vi "Main.vi"(11 "Module Admin":refnum<class "Delacor_lib_QMH_Module Admin.lvclass">) -> ()   [LabVIEW 2020, in "FileIO.lvlib"]
doc: "This template is based off of the Queued Message Handler design pattern and the Queued Message Handler project template that ships with LabVIEW.\n\nThe main difference is that the queue is private to this module and communication between modules is performed via Broadcast and Request events.\n\nRequest events are wrapped in public API methods and are handled in the Event Handling Loop (EHL) of this VI. Any module can register for Broadcast events sent by this module. The EHL generates messages based on user interface actions.\n\nThe Message Handling Loop (MHL) processes messages generated by the EHL, or by other messages. The messages are string values, so new messages can be added easily to the Message Cases case structure in the MHL. Each message cluster can also provide an optional value for Message Data, which is a variant that can be converted to whatever message-specific data is required.\n_____\nBased on Delacor QMH Project Template 5.0.0.82."
uses:
  FileIO.lvlib
  Module Data--cluster.ctl
  <vilib>/Delacor/Delacor QMH/Libraries/Message Queue_class/Delacor_lib_QMH_Message Queue.lvclass
  <vilib>/Delacor/Delacor QMH/Libraries/Message Queue_class/Delacor_lib_QMH_Enqueue Message (Single).vi
  <vilib>/ErrorRing/Error Ring.xnode
  <vilib>/Utility/error.llb/Error Cluster From Error Code.vi
  <vilib>/Delacor/Delacor QMH/Libraries/Module Admin_class/Delacor_lib_QMH_Module Admin.lvclass
  Stop Argument--cluster.ctl
  <vilib>/Utility/miscctls.llb/LVPointTypeDef.ctl
  Prepare File (Reply Payload)--cluster.ctl
  Prepare File Argument--cluster.ctl
  LabVIEW-HDF5-Tools/HDF5 Tools.lvlib
  Write to File (Reply Payload)--cluster.ctl
  Write to File Argument--cluster.ctl
panel:
  in  "Simulate MHL Error":bool
  in  "Simulate EHL Error":bool
  out "error out":errorcluster
  out "Status":string
  # "Other QMH Modules communicate with this Module via its Public API (wrappers for its Request Events).\n\nThis Module communicates with other Modules via its Broadcast Events.\nAny module that wants to get these messages, just registers for this module's Broadcast events."
  # "This template is for the Delacor Modified Queued Message Handler design pattern.\n\nSee the block diagram for more information on how to use this template."
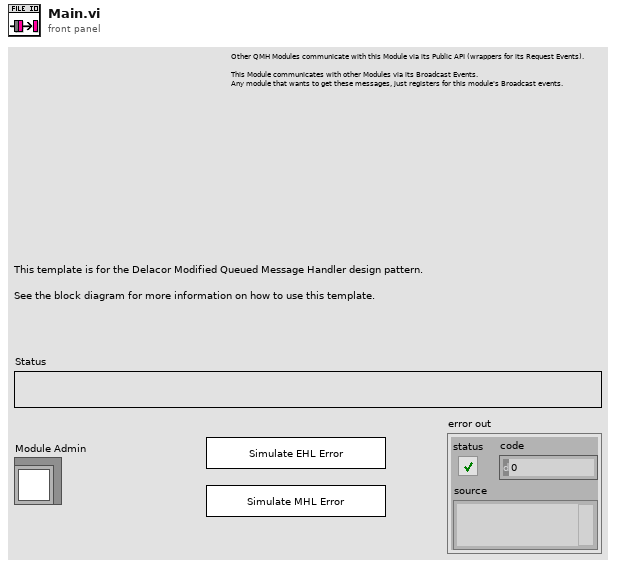
[diagram p1: front panel]
types:
  T1 = typedef "FileIO.lvlib/Request Events--cluster.ctl" = cluster{"Stop Module":refnum<user-event>, "Show Panel":refnum<user-event>, "Hide Panel":refnum<user-event>, "Get Module Execution Status":refnum<user-event>, "Show Diagram":refnum<user-event>, "Prepare File":refnum<user-event>, "Write to File":refnum<user-event>}
  T2 = typedef "FileIO.lvlib/Module Data--cluster.ctl" = cluster{"Status":string, "Data Folder":path}
  T3 = enum32{"invalid lock state", "Not Locked", "Locked (No Password)", "Password-protected"}
  T4 = typedef "FileIO.lvlib/Stop Argument--cluster.ctl" = cluster{"Origin":string, "Exit via Stop Module Req?":bool, "Wait for Module to stop?":bool}
  T5 = typedef "FileIO.lvlib/Prepare File Argument--cluster.ctl" = cluster{"name":string, "file path":path, "dims":u64[], "data":variant, "Wait Notifier":refnum<notifier>, "wait for reply":bool}
  T6 = typedef "FileIO.lvlib/Write to File Argument--cluster.ctl" = cluster{"file path":path, "indices":u64[], "data":variant, "Wait Notifier":refnum<notifier>, "wait for reply":bool}
  T7 = typedef "LVPointTypeDef.ctl" = cluster{"Horizontal":i16, "Vertical":i16}
  T8 = enum32{"Invalid", "Standard", "Closed", "Hidden", "Minimized", "Maximized"}
  T9 = typedef "FileIO.lvlib/Prepare File (Reply Payload)--cluster.ctl" = cluster{"success":bool, "file path":path, "Prepare File_error":errorcluster}
  T10 = typedef "FileIO.lvlib/Write to File (Reply Payload)--cluster.ctl" = cluster{"success":bool, "Write to File_error":errorcluster}
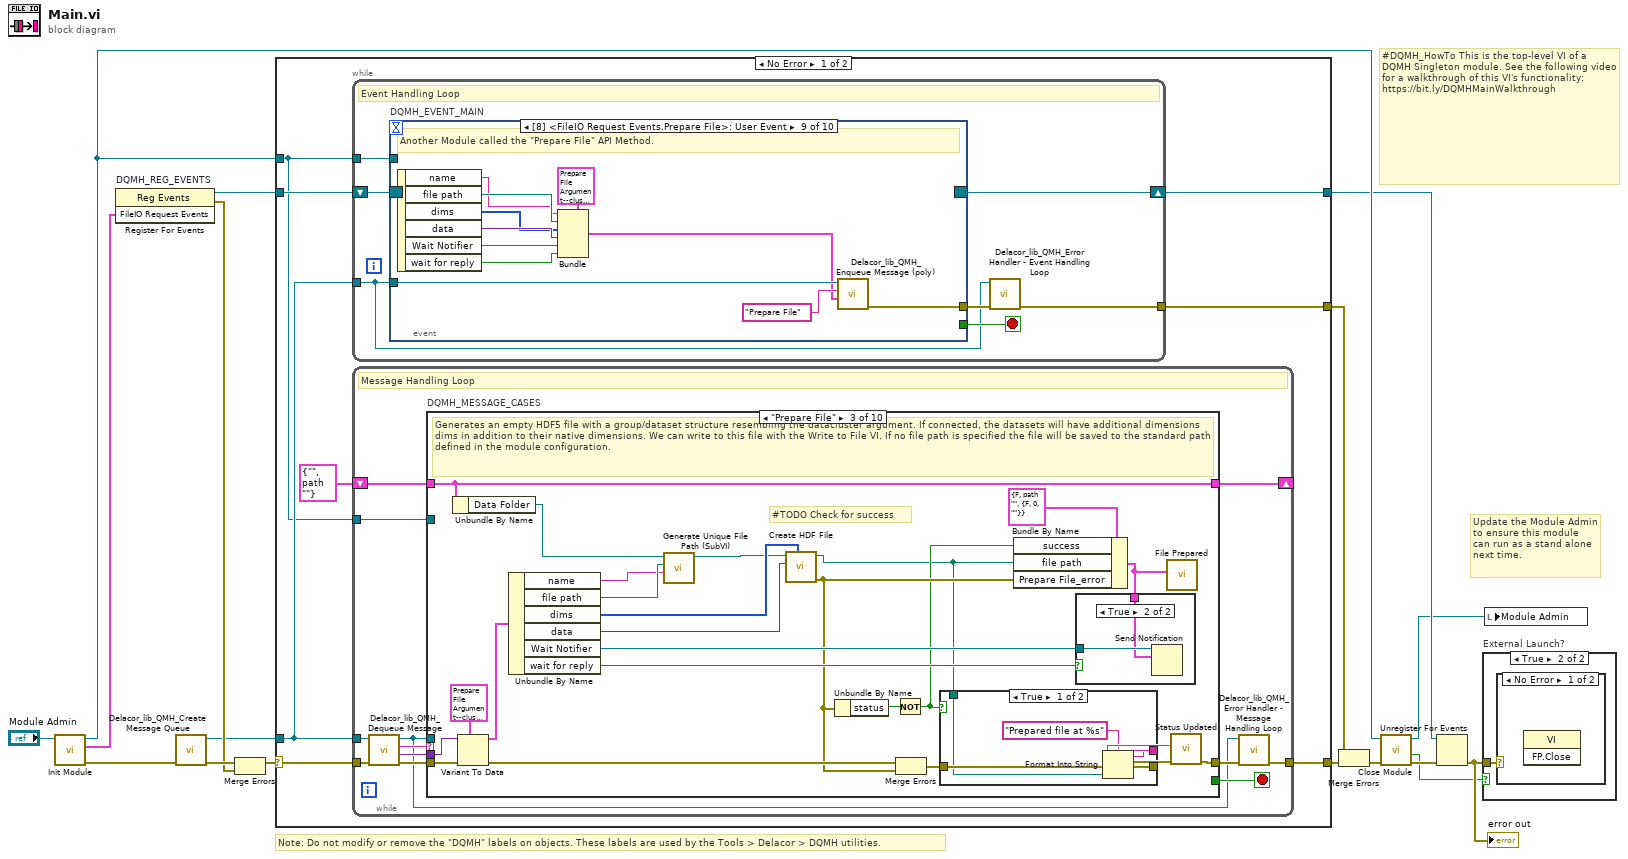
[diagram p0: block diagram]
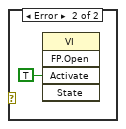
[diagram p3: hidden frame]
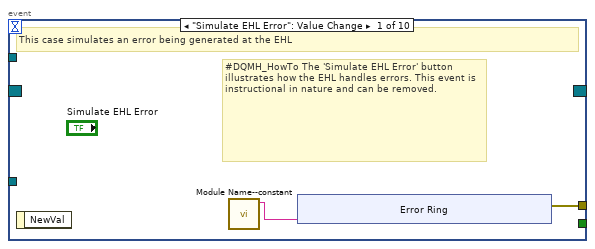
[diagram p4: hidden frame]
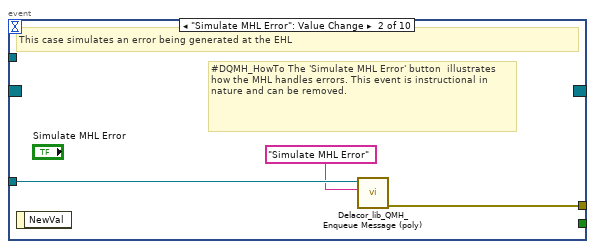
[diagram p5: hidden frame]
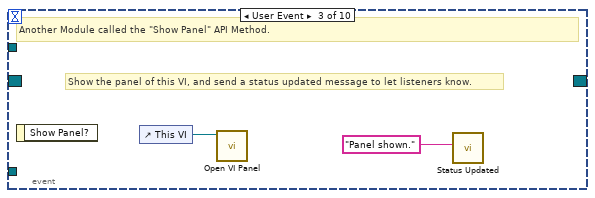
[diagram p6: hidden frame]
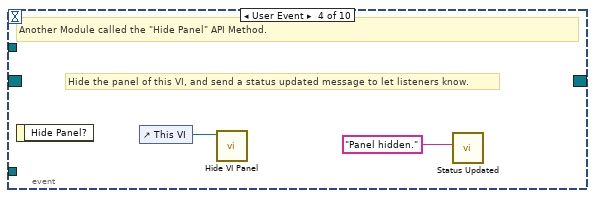
[diagram p7: hidden frame]
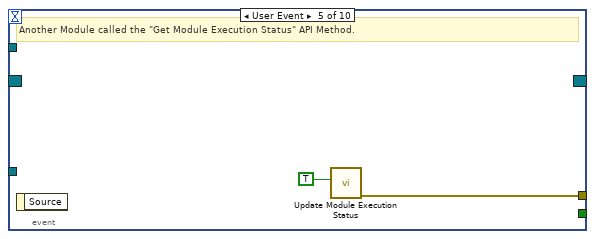
[diagram p8: hidden frame]
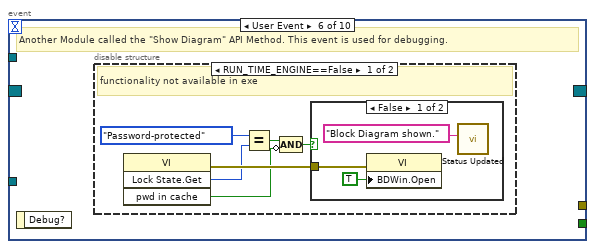
[diagram p9: hidden frame]
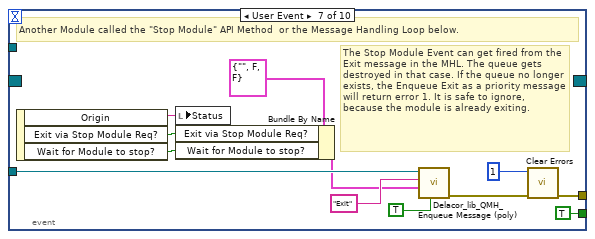
[diagram p12: hidden frame]
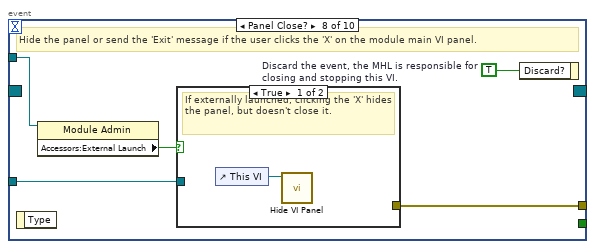
[diagram p13: hidden frame]
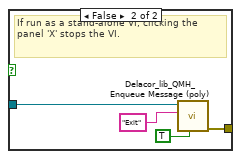
[diagram p14: hidden frame]
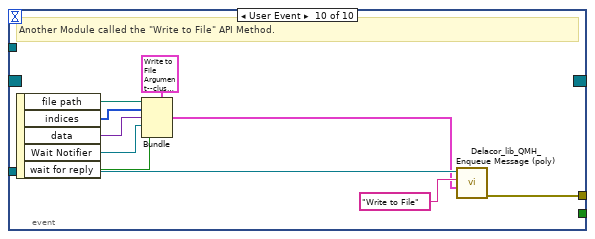
[diagram p15: hidden frame]
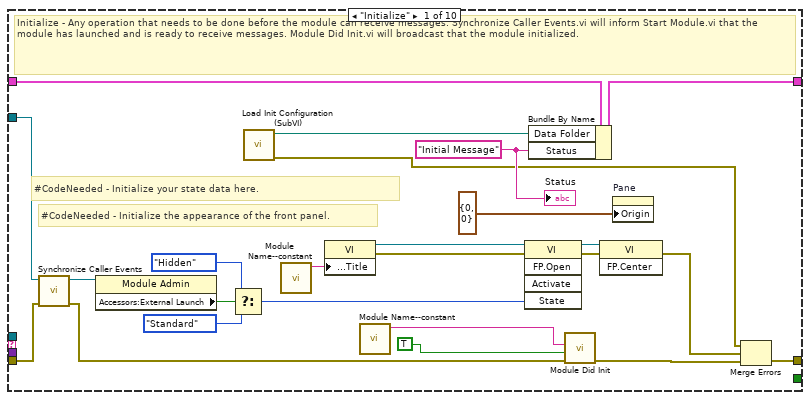
[diagram p16: hidden frame]
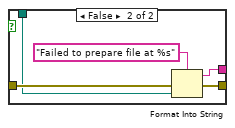
[diagram p18: hidden frame]
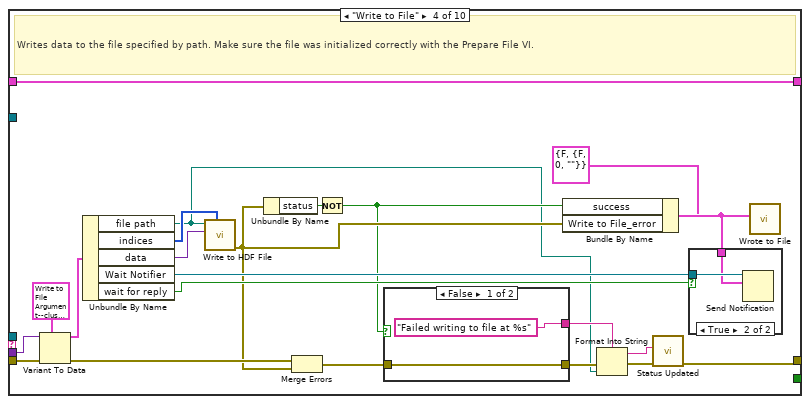
[diagram p20: hidden frame]
diagram:
  # "#DQMH_HowTo This is the top-level VI of a DQMH Singleton module. See the following video for a walkthrough of this VI's functionality: https://bit.ly/DQMHMainWalkthrough"
  # "Note: Do not modify or remove the \"DQMH\" labels on objects. These labels are used by the Tools > Delacor > DQMH utilities."
  # "Update the Module Admin to ensure this module can run as a stand alone next time."
  n1 = call "Init Module.vi"("Singleton Module Admin in"="Module Admin") -> ("error out"=w16:errorcluster, "FileIO Request Events"=w5:T1, "Singleton Module Admin out"=w8:refnum<class "Delacor_lib_QMH_Module Admin.lvclass">)  [unwired: 8 in]
  n2 = register-events "DQMH_REG_EVENTS"(w5) -> (reference out=w6:refnum<event-registration>, error out=w9:errorcluster)  [unwired: 2 in]
  n3 = call <vilib>:"Delacor_lib_QMH_Create Message Queue.vi"("error in"=w16) -> ("error out"=w11:errorcluster, "Message Queue"=w4:refnum<class "Delacor_lib_QMH_Message Queue.lvclass">)  [unwired: 9 in]
  n4 = Merge Errors(w11, w9) -> (w10:errorcluster)
  n5 = case shown="No Error" w10 {
    selector: w10 -> [w23 w270]
    tunnel: [w25 w269] -> w17
    tunnel: [w22 w275] -> w7
    tunnel: w6 -> [w20 w275]
    tunnel: w4 -> [w19 w268]
    tunnel: [w24 _] -> w14
    tunnel: w8 -> [w18 w271]
    frame No Error {
      n6 = while {
        tunnel: w19 -> [w26]
        shift-right: [w29] -> w22
        shift-left: w20 -> [w30]
        tunnel: [w31] -> w24
        tunnel: w18 -> [w27]
        stop <- w28 stop-if-true
        # "Event Handling Loop"
        n7 = event "DQMH_EVENT_MAIN" shown="[8] <FileIO Request Events.Prepare File>: User Event" {
          selector: w30 -> [_ _ _ _ _ _ _ _ _ _]
          dyn-events: [_ _ _ _ _ _ _ _ _ _] -> w29
          timeout: _ -> [_ _ _ _ _ _ _ _ _ _]
          tunnel: [_ _ _ _ _ _ TRUE ("Discard?") _ _ _] -> w28
          tunnel: w26 -> [_ w43 _ _ _ _ w67 w74 w92 w102]
          tunnel: [w34 w44 _ _ w50 _ w70 w76 w88 w93] -> w32
          tunnel: w27 -> [_ _ _ _ _ _ _ w73 _ _]
          event "Simulate EHL Error": Value Change {
            # "#DQMH_HowTo The 'Simulate EHL Error' button  illustrates how the EHL handles errors. This event is instructional in nature and can be removed."
            # "This case simulates an error being generated at the EHL"
            n8 = event-data() -> ()  [unwired: 1 in, 1 out]
            n9 = call "Module Name--constant.vi"() -> ("Module Name"=w33:string)  [unwired: 11 in]
            n10 = xnode "Error Ring"("parameter 0"=w33) -> ("error out"=w34:errorcluster)
          }
          event "Simulate MHL Error": Value Change {
            # "#DQMH_HowTo The 'Simulate MHL Error' button  illustrates how the MHL handles errors. This event is instructional in nature and can be removed."
            # "This case simulates an error being generated at the EHL"
            n11 = event-data() -> ()  [unwired: 1 in, 1 out]
            n12 = call-poly <vilib>:"Delacor_lib_QMH_Enqueue Message (poly).vi"("Message"="Simulate MHL Error", "Message Queue in"=w43) -> ("error out"=w44:errorcluster)  [unwired: 8 in, 1 out]
          }
          event User Event {
            # "Show the panel of this VI, and send a status updated message to let listeners know."
            # "Another Module called the \"Show Panel\" API Method."
            n13 = event-data() -> ()  [unwired: 1 in, 1 out]
            n14 = control-ref of="This VI"() -> (w46:refnum<vi>)
            n15 = call "Open VI Panel.vi"("VI"=w46) -> ()  [unwired: 10 in, 1 out]
            n16 = call "Status Updated.vi"("Status"="Panel shown." ("format string")) -> ()  [unwired: 10 in, 1 out]
          }
          event User Event {
            # "Hide the panel of this VI, and send a status updated message to let listeners know."
            # "Another Module called the \"Hide Panel\" API Method."
            n17 = event-data() -> ()  [unwired: 1 in, 1 out]
            n18 = control-ref of="This VI"() -> (w48:refnum<vi>)
            n19 = call "Hide VI Panel.vi"("VI"=w48) -> ()  [unwired: 10 in, 1 out]
            n20 = call "Status Updated.vi"("Status"="Panel hidden." ("format string")) -> ()  [unwired: 10 in, 1 out]
          }
          event User Event {
            # "Another Module called the \"Get Module Execution Status\" API Method."
            n21 = event-data() -> ()  [unwired: 1 in, 1 out]
            n22 = call "Update Module Execution Status.vi"("Running?"=TRUE) -> ("error out"=w50:errorcluster)  [unwired: 10 in]
          }
          event User Event {
            # "Another Module called the \"Show Diagram\" API Method. This event is used for debugging."
            n23 = event-data() -> ()  [unwired: 1 in, 1 out]
            n24 = disable-structure shown="RUN_TIME_ENGINE==False" {
              frame condition #0 (active) {
                # "functionality not available in exe"
                n25 = invoke class="VI" method="Lock State.Get"() -> (error out=w56:errorcluster, "Get Lock State"=w55:T3, "pwd in cache"=w52:bool)  [unwired: 4 in, 1 out]
                n26 = Equal?(x=T3."Password-protected", y=w55) -> (x = y?=w53:bool)
                n27 = Compound Arithmetic op=AND(w53, invert w52) -> (w51:bool)
                n28 = case shown="False" w51 {
                  tunnel: w56 -> [w59 _]
                  frame False {
                    n29 = property class="VI"(error in=w59, "BDWin.Open"=TRUE ("Block Diagram Window:Open")) -> ()  [unwired: 1 in, 2 out]
                    n30 = call "Status Updated.vi"("Status"="Block Diagram shown." ("format string")) -> ()  [unwired: 10 in, 1 out]
                  }
                  frame True {
                    # "Password-protected VI, and the password is not in the cache. Do not show the diagram."
                  }
                }
              }
              frame condition #1 {
              }
            }
          }
          event User Event {
            # "The Stop Module Event can get fired from the Exit message in the MHL. The queue gets destroyed in that case. If the queue no longer exists, the Enqueue Exit as a priority message will return error 1. It is safe to ignore, because the module is already exiting."
            # "Another Module called the \"Stop Module\" API Method  or the Message Handling Loop below."
            n31 = event-data() -> ("Origin"=w66:string, "Exit via Stop Module Req?"=w62:bool, "Wait for Module to stop?"=w61:bool)  [unwired: 1 in]
            n32 = local write "Status"(w66) -> ()
            n33 = Bundle By Name(cluster=T4 {"Origin"="", "Exit via Stop Module Req?"=FALSE, "Wait for Module to stop?"=FALSE} ("Stop Argument"), "Exit via Stop Module Req?"=w62, "Wait for Module to stop?"=w61) -> (w60:T4)
            n34 = call-poly <vilib>:"Delacor_lib_QMH_Enqueue Message (poly).vi"("Priority Message? (F)"=TRUE, "Message Data"=w60, "Message"="Exit", "Message Queue in"=w67) -> ("error out"=w71:errorcluster)  [unwired: 6 in, 1 out]
            n35 = call <vilib>:"Clear Errors.vi"("error in (no error)"=w71, "specific error code to clear (0: all)"=1) -> ("error out"=w70:errorcluster)  [unwired: 4 in, 1 out]
          }
          event Panel Close? {
            w75 = TRUE  # Discard the event, the MHL is responsible for closing and stopping this VI.
            # "Hide the panel or send the 'Exit' message if the user clicks the 'X' on the module main VI panel."
            n36 = event-data() -> ()  [unwired: 1 in, 1 out]
            n37 = property class="Module Admin"(reference=w73) -> ("Accessors:External Launch"=w72:bool)  [unwired: 1 in, 2 out]
            n38 = case shown="True" w72 {
              tunnel: w74 -> [_ w80]
              tunnel: [_ w81] -> w76
              frame True {
                # "If externally launched, clicking the 'X' hides the panel, but doesn't close it."
                n39 = control-ref of="This VI"() -> (w77:refnum<vi>)
                n40 = call "Hide VI Panel.vi"("VI"=w77) -> ()  [unwired: 10 in, 1 out]
              }
              frame False {
                # "If run as a stand-alone VI, clicking the panel 'X' stops the VI."
                n41 = call-poly <vilib>:"Delacor_lib_QMH_Enqueue Message (poly).vi"("Priority Message? (F)"=TRUE, "Message"="Exit", "Message Queue in"=w80) -> ("error out"=w81:errorcluster)  [unwired: 7 in, 1 out]
              }
            }
            n42 = event-data("Discard?"=w75) -> ()  [unwired: 1 in, 1 out]
          }
          event User Event {
            # "Another Module called the \"Prepare File\" API Method."
            n43 = event-data() -> ("name"=w82:string, "file path"=w83:path, "dims"=w84:u64[], "data"=w85:variant, "Wait Notifier"=w86:refnum<notifier>, "wait for reply"=w87:bool)  [unwired: 1 in]
            n44 = Bundle(cluster=T5 {"name"="", "file path"=path "", "dims"=[], "data"=variant, "Wait Notifier"=refnum, "wait for reply"=FALSE} ("Prepare File Argument"), "name"=w82, "file path"=w83, "dims"=w84, "data"=w85, "Wait Notifier"=w86, "wait for reply"=w87) -> (w89:T5)
            n45 = call-poly <vilib>:"Delacor_lib_QMH_Enqueue Message (poly).vi"("Message Data"=w89, "Message"="Prepare File", "Message Queue in"=w92) -> ("error out"=w88:errorcluster)  [unwired: 7 in, 1 out]
          }
          event User Event {
            # "Another Module called the \"Write to File\" API Method."
            n46 = event-data() -> ("file path"=w98:path, "indices"=w97:u64[], "data"=w96:variant, "Wait Notifier"=w95:refnum<notifier>, "wait for reply"=w94:bool)  [unwired: 1 in]
            n47 = Bundle(cluster=T6 {"file path"=path "", "indices"=[], "data"=variant, "Wait Notifier"=refnum, "wait for reply"=FALSE} ("Write to File Argument"), "file path"=w98, "indices"=w97, "data"=w96, "Wait Notifier"=w95, "wait for reply"=w94) -> (w99:T6)
            n48 = call-poly <vilib>:"Delacor_lib_QMH_Enqueue Message (poly).vi"("Message Data"=w99, "Message"="Write to File", "Message Queue in"=w102) -> ("error out"=w93:errorcluster)  [unwired: 7 in, 1 out]
          }
        }
        n49 = call-dynamic "Delacor_lib_QMH_Error Handler - Event Handling Loop.vi"("error in"=w32, "Message Queue in"=w26) -> ("dup error in"=w31:errorcluster)  [unwired: 8 in, 1 out]
      }
      n50 = while {
        tunnel: w19 -> [w105]
        shift-right: [w109] -> _
        shift-left: T2 {"Status"="", "Data Folder"=path ""} ("Data Cluster") -> [w110]
        tunnel: w23 -> [w113]
        tunnel: [w111] -> w25
        tunnel: w18 -> [w103]
        stop <- w108 stop-if-true
        # "Message Handling Loop"
        n51 = call-dynamic "Delacor_lib_QMH_Dequeue Message.vi"("error in"=w113, "Message Queue in"=w105) -> ("error out"=w112:errorcluster, "Message Data"=w106:variant, "Message"=w107:string, "Message Queue out"=w104:refnum<class "Delacor_lib_QMH_Message Queue.lvclass">)  [unwired: 6 in]
        n52 = case "DQMH_MESSAGE_CASES" shown="\"Prepare File\"" w107 {
          selector: w107 -> [_ _ _ _ _ _ _ _ _ w255]
          tunnel: w104 -> [_ _ _ _ _ _ _ w225 w247 _]
          tunnel: w112 -> [w136 w140 w164 w198 w207 w209 w214 w232 w253 w257]
          tunnel: [w117 w140 w148 w178 w206 w209 w213 w228 w250 w258] -> w114
          tunnel: w110 -> [w125 w139 w145 w197 w205 w208 w211 w227 w246 w256]
          tunnel: [w124 w139 w145 w197 w205 w208 w211 w227 w246 w256] -> w109
          tunnel: [_ _ _ _ _ _ _ _ w245 _] -> w108
          tunnel: w106 -> [_ _ w162 w195 _ _ _ w226 w244 _]
          tunnel: w103 -> [w126 _ _ _ _ _ _ w224 w239 _]
          frame "Initialize" {
            w119 = "Initial Message" ("Initial Message")
            # "#CodeNeeded - Initialize the appearance of the front panel."
            # "#CodeNeeded - Initialize your state data here."
            # "Initialize - Any operation that needs to be done before the module can receive messages. Synchronize Caller Events.vi will inform Start Module.vi that the module has launched and is ready to receive messages. Module Did Init.vi will broadcast that the module initialized."
            n53 = call "Synchronize Caller Events.vi"("error in (no error)"=w136, "Singleton Module Admin in"=w126) -> ("error out"=w135:errorcluster, "Singleton Module Admin out"=w121:refnum<class "Delacor_lib_QMH_Module Admin.lvclass">)  [unwired: 8 in]
            n54 = property class="Module Admin"(reference=w121) -> ("Accessors:External Launch"=w130:bool)  [unwired: 1 in, 2 out]
            n55 = Select(t=T8."Hidden" ("State"), s=w130, f=T8."Standard" ("State")) -> (s? t:f=w127:T8)
            n56 = call "Load Init Configuration (SubVI).vi"() -> ("error out"=w115:errorcluster, "datafolder"=w118:path)  [unwired: 10 in]
            n57 = call "Module Name--constant.vi"() -> ("Module Name"=w133:string)  [unwired: 11 in]
            n58 = property class="VI"("Front Panel.Title"=w133) -> (reference out=w132:refnum<vi>, error out=w138:errorcluster)  [unwired: 2 in]
            n59 = call "Module Name--constant.vi"() -> ("Module Name"=w122:string)  [unwired: 11 in]
            n60 = invoke class="VI" method="FP.Open"(reference=w132, error in=w138, "State"=w127) -> (reference out=w131:refnum<vi>, error out=w137:errorcluster)  [unwired: 2 in, 3 out]
            n61 = Bundle By Name(cluster=w125, "Data Folder"=w118, "Status"=w119) -> (w124:T2)
            n62 = call "Module Did Init.vi"("error in (no error)"=w135, "Initialized?"=TRUE, "Origin"=w122) -> ("error out"=w134:errorcluster)  [unwired: 8 in]
            n63 = invoke class="VI" method="FP.Center"(reference=w131, error in=w137) -> (error out=w116:errorcluster)  [unwired: 1 in, 2 out]
            n64 = property on="Pane" class="Pane"("Origin"=T7 {"Horizontal"=0, "Vertical"=0}) -> ()  [unwired: 2 in, 2 out]
            n65 = Merge Errors(w115, w116, w134) -> (w117:errorcluster)
            "Status" <- w119
          }
          frame "--- Module Specific ---" {
            # "Separator -- The following cases handle messages specific to this Module."
          }
          frame "Prepare File" {
            # "#TODO Check for success"
            # "Generates an empty HDF5 file with a group/dataset structure resembling the datacluster argument. If connected, the datasets will have additional dimensions dims in addition to their native dimensions. We can write to this file with the Write to File VI. If no file path is specified the file will be saved to the standard path defined in the module configuration."
            n66 = Unbundle By Name(w145) -> ("Data Folder"=w144:path)
            n67 = Variant To Data(error in=w164, type=T5 {"name"="", "file path"=path "", "dims"=[], "data"=variant, "Wait Notifier"=refnum, "wait for reply"=FALSE} ("Prepare File Argument"), Variant=w162) -> (data=w160:T5, error out=w163:errorcluster)
            n68 = Unbundle By Name(w160) -> ("name"=w141:string, "file path"=w142:path, "dims"=w154:u64[], "data"=w155:variant, "Wait Notifier"=w159:refnum<notifier>, "wait for reply"=w158:bool)
            n69 = call "Generate Unique File Path (SubVI).vi"("Measurement Name"=w141, "file path"=w142, "Data Folder"=w144) -> ("appended path"=w143:path)  [unwired: 7 in, 1 out]
            n70 = call "Create HDF File.vi"("Dims"=w154, "variant"=w155, "path"=w143) -> ("error out"=w153:errorcluster, "path out"=w147:path)  [unwired: 6 in, 1 out]
            n71 = Unbundle By Name(w153) -> ("status"=w152:bool)
            n72 = Not(x=w152) -> (.not. x?=w149:bool)
            n73 = Merge Errors(w163, w153) -> (w151:errorcluster)
            n74 = case shown="True" w149 {
              tunnel: w151 -> [w168 w173]
              tunnel: [w167 w172] -> w150
              tunnel: w147 -> [w166 w171]
              tunnel: [w165 w170] -> w146
              frame True {
                n75 = Format Into String(format string="Prepared file at %s", error in=w168, w166) -> (resulting string=w165:string, error out=w167:errorcluster)  [unwired: 1 in]
              }
              frame False {
                n76 = Format Into String(format string="Failed to prepare file at %s", error in=w173, w171) -> (resulting string=w170:string, error out=w172:errorcluster)  [unwired: 1 in]
              }
            }
            n77 = Bundle By Name(cluster=T9 {"success"=FALSE, "file path"=path "", "Prepare File_error"={"status"=FALSE, "code"=0, "source"=""}} ("Prepare File (Reply Payload)"), "success"=w149, "file path"=w147, "Prepare File_error"=w153) -> (w157:T9)
            n78 = case shown="True" w158 {
              tunnel: w159 -> [_ w176]
              tunnel: w157 -> [_ w175]
              frame False {
              }
              frame True {
                n79 = Send Notification(notification=w175, notifier=w176) -> ()  [unwired: 1 in, 2 out]
              }
            }
            n80 = call "File Prepared.vi"("Reply Payload"=w157) -> ()  [unwired: 10 in, 1 out]
            n81 = call "Status Updated.vi"("error in (no error)"=w150, "Status"=w146) -> ("error out"=w148:errorcluster)  [unwired: 9 in]
          }
          frame "Write to File" {
            # "Writes data to the file specified by path. Make sure the file was initialized correctly with the Prepare File VI."
            n82 = Variant To Data(error in=w198, type=T6 {"file path"=path "", "indices"=[], "data"=variant, "Wait Notifier"=refnum, "wait for reply"=FALSE} ("Write to File Argument"), Variant=w195) -> (data=w193:T6, error out=w196:errorcluster)
            n83 = Unbundle By Name(w193) -> ("file path"=w179:path, "indices"=w187:u64[], "data"=w188:variant, "Wait Notifier"=w192:refnum<notifier>, "wait for reply"=w191:bool)
            n84 = call "Write to HDF File.vi"("indices"=w187, "variant"=w188, "path"=w179) -> ("error out"=w186:errorcluster)  [unwired: 8 in]
            n85 = Unbundle By Name(w186) -> ("status"=w185:bool)
            n86 = Merge Errors(w196, w186) -> (w183:errorcluster)
            n87 = Not(x=w185) -> (.not. x?=w184:bool)
            n88 = case shown="False" w184 {
              tunnel: w183 -> [w199 w202]
              tunnel: [w199 w202] -> w182
              tunnel: ["Failed writing to file at %s" "Wrote to file at %s"] -> w180
              frame False {
              }
              frame True {
              }
            }
            n89 = Bundle By Name(cluster=T10 {"success"=FALSE, "Write to File_error"={"status"=FALSE, "code"=0, "source"=""}} ("Write to File (Reply Payload)"), "success"=w184, "Write to File_error"=w186) -> (w190:T10)
            n90 = Format Into String(format string=w180, error in=w182, w179) -> (resulting string=w177:string, error out=w181:errorcluster)  [unwired: 1 in]
            n91 = call "Status Updated.vi"("error in (no error)"=w181, "Status"=w177) -> ("error out"=w178:errorcluster)  [unwired: 9 in]
            n92 = case shown="True" w191 {
              tunnel: w192 -> [_ w204]
              tunnel: w190 -> [_ w203]
              frame False {
              }
              frame True {
                n93 = Send Notification(notification=w203, notifier=w204) -> ()  [unwired: 1 in, 2 out]
              }
            }
            n94 = call "Wrote to File.vi"("Reply Payload"=w190) -> ()  [unwired: 10 in, 1 out]
          }
          frame "---Copy This Frame---" {
            # "Duplicate this frame when creating new messages.  Change this comment in the duplicated frame to describe this message."
            n95 = Merge Errors(w207) -> (w206:errorcluster)
          }
          frame "--- Exit and Error Handling---" {
            # "Separator - The following cases handle errors and exit messages."
          }
          frame "Simulate MHL Error" {
            # "#DQMH_HowTo The 'Simulate MHL Error' button  illustrates how the MHL handles errors. This event is instructional in nature and can be removed."
            # "Simulate an error occurring at the MHL"
            n96 = call "Module Name--constant.vi"() -> ("Module Name"=w210:string)  [unwired: 11 in]
            n97 = xnode "Error Ring"("parameter 0"=w210) -> ("error out"=w212:errorcluster)
            n98 = Merge Errors(w214, w212) -> (w213:errorcluster)
          }
          frame "Error" {
            # "#CodeRecommended - If you ever change the name of this \"Error\" message, you'll need to update the name in the Check Loop Error.vi as well."
            # "#CodeRecommended - If the module is running in standalone mode (External Launch = FALSE), this code will pop up an error dialog and call the 'Exit' message if an error occurs. Add more fine-grained error handling here."
            # "Error - Check the error message data and respond accordingly. This message is sent by the \"Error Handler\" VIs at the end of each loop in this application."
            n99 = property class="Module Admin"(reference=w224) -> ("Accessors:External Launch"=w223:bool)  [unwired: 1 in, 2 out]
            n100 = Variant To Data(error in=w232, type=errorcluster {"status"=FALSE, "code"=0, "source"=""} ("error constant"), Variant=w226) -> (data=w233:errorcluster, error out=w230:errorcluster)
            n101 = call "Module Name--constant.vi"() -> ("Module Name"=w222:string)  [unwired: 11 in]
            n102 = call "Error Reported.vi"("Additional Information"=w222, "Error"=w233) -> ()  [unwired: 9 in, 1 out]
            n103 = case shown="False" w223 {
              tunnel: [w238 _] -> w229
              tunnel: w225 -> [w236 _]
              tunnel: w233 -> [w237 _]
              frame False {
                # "If the module is running standalone, then pop up an error dialog and call the \"Exit\" message."
                n104 = call <vilib>:"Simple Error Handler.vi"("error in (no error)"=w237) -> ()  [unwired: 4 in, 5 out]
                n105 = call-poly <vilib>:"Delacor_lib_QMH_Enqueue Message (poly).vi"("Priority Message? (F)"=TRUE, "Message"="Exit", "Message Queue in"=w236) -> ("error out"=w238:errorcluster)  [unwired: 7 in, 1 out]
              }
              frame True {
                # "If the module was launched externally, calling the Error Reported broadcast VI is the only action performed by the \"Error\" message. The module's caller can then process the error appropriately."
              }
            }
            n106 = Merge Errors(w230, w229) -> (w228:errorcluster)
            n107 = local write "error out"(w228) -> ()
          }
          frame "Exit" {
            w243 = 91  # 91: not all Exit messages will have an argument
            w245 = TRUE  # Stop the VI
            # "Release the message queue reference"
            # "#CodeNeeded - Add any required cleanup code here"
            # "Exit - Exit the application."
            n108 = Variant To Data(error in=w253, type=T4 {"Origin"="", "Exit via Stop Module Req?"=FALSE, "Wait for Module to stop?"=FALSE} ("Stop Argument"), Variant=w244) -> (data=w241:T4, error out=w249:errorcluster)
            n109 = call <vilib>:"Clear Errors.vi"("error in (no error)"=w249, "specific error code to clear (0: all)"=w243) -> ("error out"=w252:errorcluster)  [unwired: 4 in, 1 out]
            n110 = control-ref of="This VI"() -> (w240:refnum<vi>)
            n111 = call-dynamic "Delacor_lib_QMH_Release Message Queue.vi"("error in"=w252, "Message Queue"=w247) -> ("error out"=w251:errorcluster)  [unwired: 9 in]
            n112 = call "Handle Exit.vi"("Stop Argument"=w241, "Admin in"=w239, "VI reference"=w240) -> ("error out"=w248:errorcluster)  [unwired: 7 in, 1 out]
            n113 = Merge Errors(w251, w248) -> (w250:errorcluster)
          }
          frame Default {
            # "'Default' case only runs if there is a message that isn't defined in any of the other cases.  Output a programming error."
            n114 = call "Module Name--constant.vi"() -> ("Module Name"=w254:string)  [unwired: 11 in]
            n115 = xnode "Error Ring"("parameter 0"=w255, "parameter 1"=w254) -> ("error out"=w259:errorcluster)
            n116 = Merge Errors(w257, w259) -> (w258:errorcluster)
          }
        }
        n117 = call-dynamic "Delacor_lib_QMH_Error Handler - Message Handling Loop.vi"("error in"=w114, "Message Queue in"=w104) -> ("dup error in"=w111:errorcluster)  [unwired: 8 in, 1 out]
      }
    }
    frame Error {
      # "Synchronize Caller Events.vi will inform Start Module.vi that the module has launched and will let the code calling Start Module.vi register for broadcasts and would permit the caller receive the broadcast that an error occurred at launch time."
      n118 = call-dynamic "Delacor_lib_QMH_Release Message Queue.vi"("error in"=w270, "Message Queue"=w268) -> ("error out"=w269:errorcluster)  [unwired: 9 in]
      n119 = call "Synchronize Caller Events.vi"("Singleton Module Admin in"=w271) -> ("error out"=w276:errorcluster)  [unwired: 9 in, 1 out]
      n120 = call "Module Name--constant.vi"() -> ("Module Name"=w274:string)  [unwired: 11 in]
      n121 = Format Into String(format string="An error occurred during initialization. %s is no longer running.", w274) -> (resulting string=w272:string)  [unwired: 2 in, 1 out]
      n122 = Merge Errors(w269, w276) -> (w277:errorcluster)
      n123 = call "Error Reported.vi"("Additional Information"=w272, "Error"=w277) -> ()  [unwired: 9 in, 1 out]
    }
  }
  n124 = Merge Errors(w14, w17) -> (w13:errorcluster)
  n125 = call "Close Module.vi"("error in (no error)"=w13, "Module Admin in"=w8) -> ("error out"=w15:errorcluster, "External Launch"=w1:bool, "Module Admin out"=w2:refnum<class "Delacor_lib_QMH_Module Admin.lvclass">)  [unwired: 7 in]
  n126 = Unregister For Events(event registration refnum=w7, error in=w15) -> (error out=w12:errorcluster)
  "error out" <- w12
  n127 = case "External Launch?" shown="True" w1 {
    tunnel: w12 -> [_ w278]
    frame False {
    }
    frame True {
      n128 = case shown="No Error" w278 {
        frame No Error {
          n129 = invoke class="VI" method="FP.Close"() -> ()  [unwired: 3 in, 3 out]
        }
        frame Error {
          n130 = invoke class="VI" method="FP.Open"("Activate"=TRUE ("Activate?")) -> ()  [unwired: 4 in, 5 out]
        }
      }
    }
  }
  n131 = local write "Module Admin"(w2) -> ()
